vi "radio_check_response.vi"(8 "error in":errorcluster, 11 "VISA in":refnum<visa-resource-name>) -> (0 "error out":errorcluster, 1 "ok":bool, 2 "read buffer":string, 3 "VISA out":refnum<visa-resource-name>)   [LabVIEW 2011]
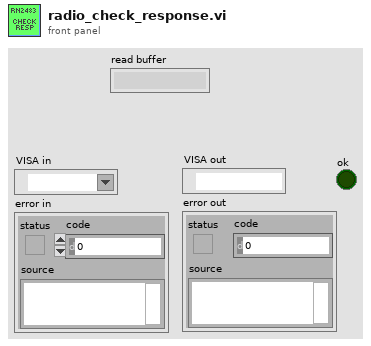
[diagram p1: front panel]
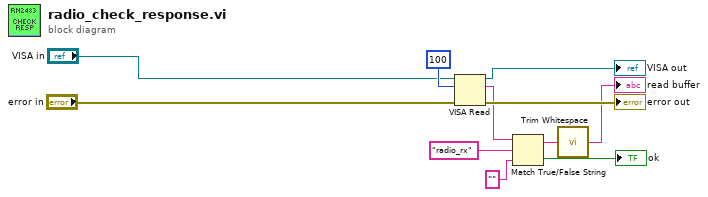
[diagram p0: block diagram]
diagram:
  n1 = VISA Read(VISA resource name="VISA in", byte count=u32 100, error in (no error)="error in") -> (VISA resource name out=→"VISA out":refnum<visa-resource-name>, read buffer=w6:string, error out=→"error out":errorcluster)  [unwired: 1 out]
  n2 = Match True/False String(2:"" ("false string"), 3:"radio_rx" ("y"), 4:w6) -> (0:→"ok":bool, 1:w2:string)
  n3 = call <vilib>:"Trim Whitespace.vi"("string"=w2) -> ("trimmed string"=→"read buffer":string)  [unwired: 1 in]
